vi "T7MOD_Write_UINT16_Register.vi"(6 "Timeout":u32=10000, 7 "UINT16 to Write":u16, 8 "error in":errorcluster, 9 "LabJack UINT16 Register":i32=55110, 10 "Remote Port":u16=502, 11 "Remote IP Address":string="192.168.1.15") -> (0 "error out":errorcluster, 1 "Written At":timestamp)   [LabVIEW 2018]
panel:
  # "Input"
  # "TCP Parameters"
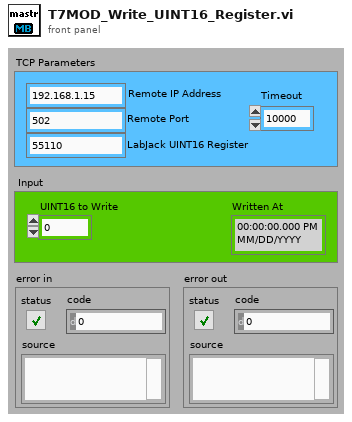
[diagram p1: front panel]
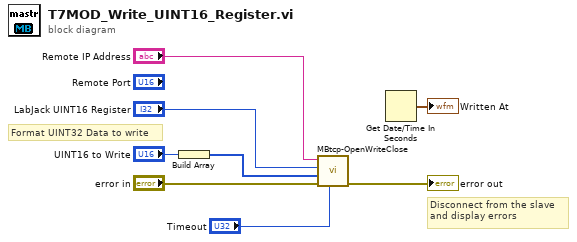
[diagram p0: block diagram]
diagram:
  # "Format UINT32 Data to write"
  # "Disconnect from the slave\nand display errors"
  n1 = Build Array("UINT16 to Write") -> (w6:u16[])
  n2 = call "MBtcp-OpenWriteClose.vi"("Timeout (900)"="Timeout", "error in (no error)"="error in", "Values"=w6, "RegisterAddr"="LabJack UINT16 Register", "IP Address(:port)"="Remote IP Address") -> ("error out"=→"error out":errorcluster)  [unwired: 6 in]
  n3 = Get Date/Time In Seconds() -> (seconds since 1Jan1904=→"Written At":timestamp)
